vi "Msg.Q.Obtain.vi"(8 "Error (in)":errorcluster, 11 "Queue Name (in)":string) -> (0 "Error (out)":errorcluster, 3 "Msg.Q.Ref":T1)   [LabVIEW 2023, in "MessagingModule.lvlib"]
doc: "This VI is used to obtain a queue of message and data."
uses:
  Msg.Q.Ref.ctl
  Msg.Data.ctl
  MessagingModule.lvlib
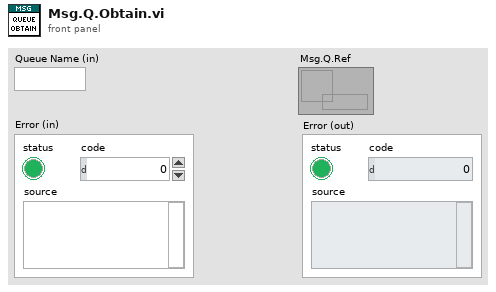
[diagram p1: front panel]
types:
  T1 = typedef "MessagingModule.lvlib/Msg.Q.Ref.ctl" = refnum<queue>
  T2 = typedef "MessagingModule.lvlib/Msg.Data.ctl" = cluster{"Message":string, "Data":variant}
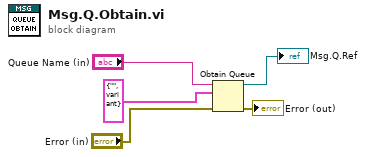
[diagram p0: block diagram]
diagram:
  n1 = Obtain Queue(name (unnamed)="Queue Name (in)", element data type=T2 {"Message"="", "Data"=variant} ("Msg.Q.Data"), error in (no error)="Error (in)") -> (queue out=→"Msg.Q.Ref":refnum<queue>, error out=→"Error (out)":errorcluster)  [unwired: 2 in, 1 out]
